vi "readLightBarriersNew.vi"() -> (0 "light barriers":bool[](array[boolean]), 1 "error out":errorcluster)   [LabVIEW 2012]
uses:
  GlobalArduinoNew.vi
  <vilib>/LabVIEW Interface for Arduino/LabVIEW Interface for Arduino.lvlib
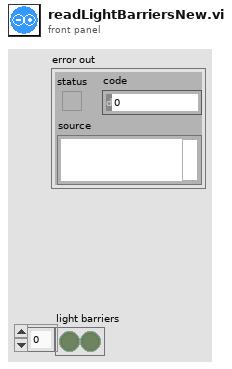
[diagram p1: front panel]
types:
  T1 = typedef "Semaphore RefNum" = refnum<k1>
  T2 = typedef "LabVIEW Interface for Arduino.lvlib/Arduino Resource.ctl" = cluster{"VISA resource":refnum<visa-resource-name>, "Board Type":T3, "Connection Type":enum8{"USB / Serial"}, "Bytes Per Packet (15)":u8}
  T3 = typedef "LabVIEW Interface for Arduino.lvlib/Board Type.ctl" = enum16{"Uno", "Dimuelanove w/Atmega 328", "Mega 2560"}
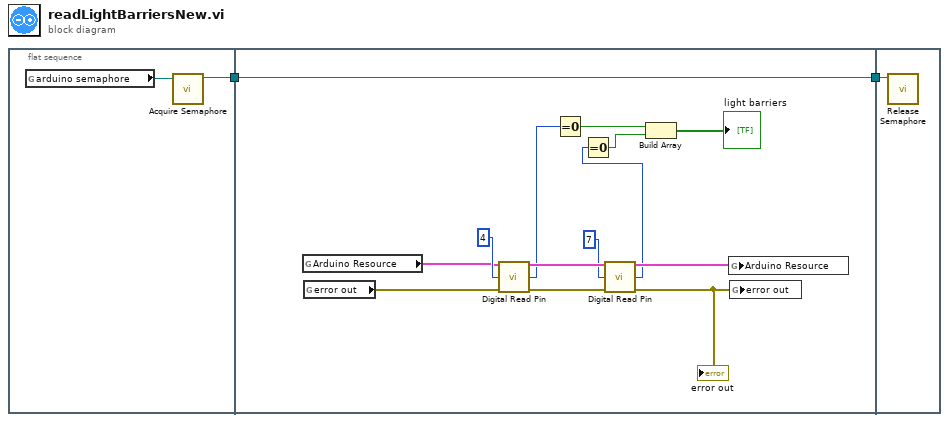
[diagram p0: block diagram]
diagram:
  n1 = flat-sequence {
    tunnel: [w3] -> w2
    tunnel: w2 -> [w5]
    tunnel: [w5] -> w1
    tunnel: w1 -> [w19]
    frame #0 {
      n2 = global read "GlobalArduinoNew.vi" "arduino semaphore"() -> (w4:T1)
      n3 = call <vilib>:"Acquire Semaphore.vi"("semaphore"=w4) -> ("semaphore out"=w3:T1)  [unwired: 4 in, 2 out]
    }
    frame #1 {
      n4 = global read "GlobalArduinoNew.vi" "Arduino Resource"() -> (w14:T2)
      n5 = global read "GlobalArduinoNew.vi" "error out"() -> (w13:errorcluster)
      n6 = call <vilib>:"Digital Read Pin.vi"("Arduino Resource"=w14, "Digital I/O Pin (0)"=u8 4, "error in"=w13) -> ("Arduino Resource"=w17:T2, "Value"=w8:u8, "error out"=w16:errorcluster)  [unwired: 10 in]
      n7 = Equal To 0?(x=w8) -> (x = 0?=w9:bool)
      n8 = call <vilib>:"Digital Read Pin.vi"("Arduino Resource"=w17, "Digital I/O Pin (0)"=u8 7, "error in"=w16) -> ("Arduino Resource"=w12:T2, "Value"=w6:u8, "error out"=w11:errorcluster)  [unwired: 10 in]
      "error out" <- w11
      n9 = Equal To 0?(x=w6) -> (x = 0?=w7:bool)
      n10 = Build Array(w9, w7) -> (→"light barriers":bool[])
      n11 = global write "GlobalArduinoNew.vi" "Arduino Resource"(w12) -> ()
      n12 = global write "GlobalArduinoNew.vi" "error out"(w11) -> ()
    }
    frame #2 {
      n13 = call <vilib>:"Release Semaphore.vi"("semaphore"=w19) -> ()  [unwired: 5 in, 2 out]
    }
  }
